vi "ModbusTxTimestampFIFO.vi"   [LabVIEW 2016]
uses:
  <vilib>/rvi/Emulation/niFpgaGetClockAttributes.vi
  <vilib>/rvi/Emulation/niFpgaSctlEmulationGetInTimedLoop.vi
  <vilib>/rvi/Emulation/niFpgaEmulationReportErrorSimple.vi
  <vilib>/rvi/Emulation/niFpgaCriticalErrorInLSC.vi
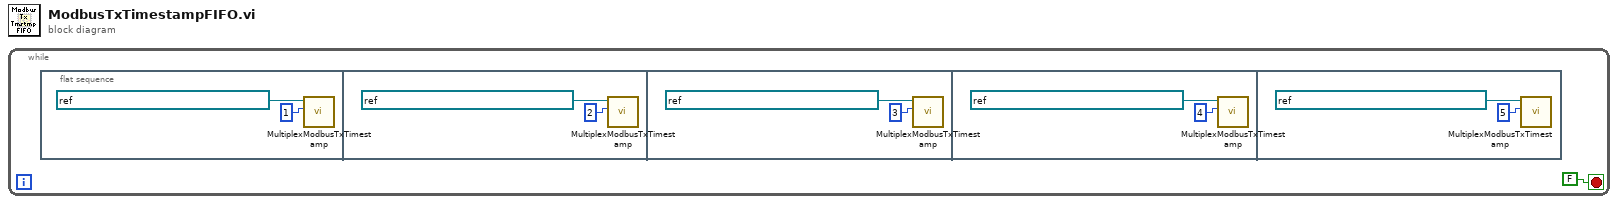
[diagram p0: block diagram]
diagram:
  n1 = while {
    stop <- FALSE stop-if-true
    n2 = flat-sequence {
      frame #0 {
        n3 = call "MultiplexModbusTxTimestamp.vi"("ID"=u64 1, "InputFIFO"=refnum<k21> "ModbusSubnetATxTimestampFIFO") -> ()  [unwired: 10 in]
      }
      frame #1 {
        n4 = call "MultiplexModbusTxTimestamp.vi"("ID"=u64 2, "InputFIFO"=refnum<k21> "ModbusSubnetBTxTimestampFIFO") -> ()  [unwired: 10 in]
      }
      frame #2 {
        n5 = call "MultiplexModbusTxTimestamp.vi"("ID"=u64 3, "InputFIFO"=refnum<k21> "ModbusSubnetCTxTimestampFIFO") -> ()  [unwired: 10 in]
      }
      frame #3 {
        n6 = call "MultiplexModbusTxTimestamp.vi"("ID"=u64 4, "InputFIFO"=refnum<k21> "ModbusSubnetDTxTimestampFIFO") -> ()  [unwired: 10 in]
      }
      frame #4 {
        n7 = call "MultiplexModbusTxTimestamp.vi"("ID"=u64 5, "InputFIFO"=refnum<k21> "ModbusSubnetETxTimestampFIFO") -> ()  [unwired: 10 in]
      }
    }
  }
